vi "Stabilization Insulated Sphere FGV.vi"(11 "Stabilization Value In":dbl format="%#_13g") -> (3 "Stabilization Array Out":dbl[](array[numeric]))   [LabVIEW 2013]
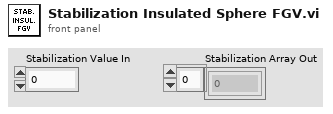
[diagram p1: front panel]
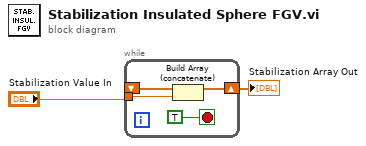
[diagram p0: block diagram]
diagram:
  n1 = while {
    tunnel: "Stabilization Value In" -> [w6]
    shift-right: [w4] -> w1
    shift-left: _ -> [w5]
    stop <- TRUE stop-if-true
    n2 = Build Array (concatenate)(w5, w6) -> (w4:dbl[])
  }
  "Stabilization Array Out" <- w1
